vi "FRCts20_WebMethods_Events_Events_GET.vi"(7 "httpRequestID":u32, 11 "view":string) -> ()   [LabVIEW 2014]
doc: "<B>GET</B> on the specified <B>competition</B> resource\n\n<B>Default Return:</B> <B>competition</B> information and list of contained divisions\n\n<B>query =</B> info - Returns only <B>competition</B> information\n stats - Returns statistics for <B>competition</B>\n images - Returns .png and .jpeg images for <B>competition</B>\n videos - Returns .wmv videos for <B>competition</B>\n\nhttp://<server address>:<port>/FRCts/competition/<B>competition</B>"
uses:
  FRCts20_WebMethods.lvlib
  Backend/source/VI Source/FRCts20_Backend_API/FRCts20_Backend_API.lvlib
  <vilib>/wsapi/NI_WebServices.lvlib
  ESP Engine/source/VI Source/FRCts20_EspEngine.lvlib
  Web Method Public Interface/FRCts20_WebMethods_ctl_teamIdentifier.ctl
  Web Method Public Interface/FRCts20_WebMethods_ctl_singleEvent.ctl
  Web Method Public Interface/FRCts20_WebMethods_ctl_events.ctl
  Backend/source/VI Source/FRCts20_Backend_API/FRCts20_Backend_API_Command_Division.ctl
  Backend/source/VI Source/FRCts20_Backend_API/FRCts20_Backend_API_Event.vi
panel:
  in  "events":string
  out "error out":errorcluster
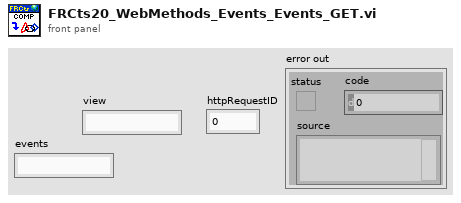
[diagram p1: front panel]
types:
  T1 = typedef "FRCts20_Backend_API.lvlib/FRCts20_Backend_API_Command_Division.ctl" = string
  T2 = typedef "FRCts20_WebMethods.lvlib/FRCts20_WebMethods_ctl_events.ctl" = cluster{"Live Events":cluster{"Team":T3[], "Issue Count":i32, "Location":string, "Start Date ":timestamp}[], "Non Live Events":T4[]}
  T3 = typedef "FRCts20_WebMethods.lvlib/FRCts20_WebMethods_ctl_teamIdentifier.ctl" = cluster{"Team Nickname":string, "Team Number ":u32, "UniqueId":u32}
  T4 = typedef "FRCts20_WebMethods.lvlib/FRCts20_WebMethods_ctl_singleEvent.ctl" = cluster{"Team":T3[], "Issue Count":i32, "Location":string, "Start Date ":timestamp}
  T5 = typedef "FRCts20_WebMethods.lvlib/FRCts20_WebMethods_ctl_returntype.ctl" = string
  T6 = typedef "FRCts20_EspEngine.lvlib/FRCts20_EspEngine_Universe.ctl" = cluster{"TeamsListLength":i16, "Teams":T7[], "LiveEventListLength":i16, "LiveEvents":T12[], "NonLiveEventListLength":i16, "NonLiveEvents":T12[], "OpenIssueCount":i16, "NotFoundStatus":bool}
  T7 = typedef "FRCts20_EspEngine.lvlib/FRCts20_EspEngine_Team.ctl" = cluster{"Team":T8, "RequestListLength":i16, "Requests":T10[]}
  T8 = typedef "FRCts20_WebMethods.lvlib/FRCts20_WebMethods_ctl_singleTeam.ctl" = cluster{"Events":string[], "Robot Name":string, "Kinect":bool, "Vision":bool, "Can":bool, "Tags":string, "Avatar URL":string, "Team":T3, "SWType":T9}
  T9 = typedef "FRCts20_Backend_API.lvlib/FRCts20_Backend_API_SW.ctl" = string
  T10 = typedef "FRCts20_WebMethods.lvlib/FRCts20_WebMethods_ctl_request.ctl" = cluster{"Event":string, "Description":string, "Status":T11, "Open Date":string, "Last Update":string, "Close Date":string, "UniqueId":i32, "Team":cluster{"Team Nickname":string, "Team Number ":i32, "UniqueId":i32}, "Comments":cluster{"Request Number":dbl, "Text":string, "Author":string, "IsSolution":bool, "Team":cluster{"Team Nickname":string, "Team Identifier ":dbl}, "UniqueId":i32}[]}
  T11 = typedef "FRCts20_Backend_API.lvlib/FRCts20_Backend_API_Status.ctl" = enum16{"Open", "In Work", "Closed"}
  T12 = typedef "FRCts20_EspEngine.lvlib/FRCts20_EspEngine_Event.ctl" = cluster{"Single Event":T4, "EventOpenIssueCount":i16, "Requests":cluster{"RequestId":i32, "Request Description":string, "Team Number":i32}[], "ClosedRequests":cluster{"RequestId":i32, "Request Description":string, "Team Number":i32}[], "NotFoundStatus":bool}
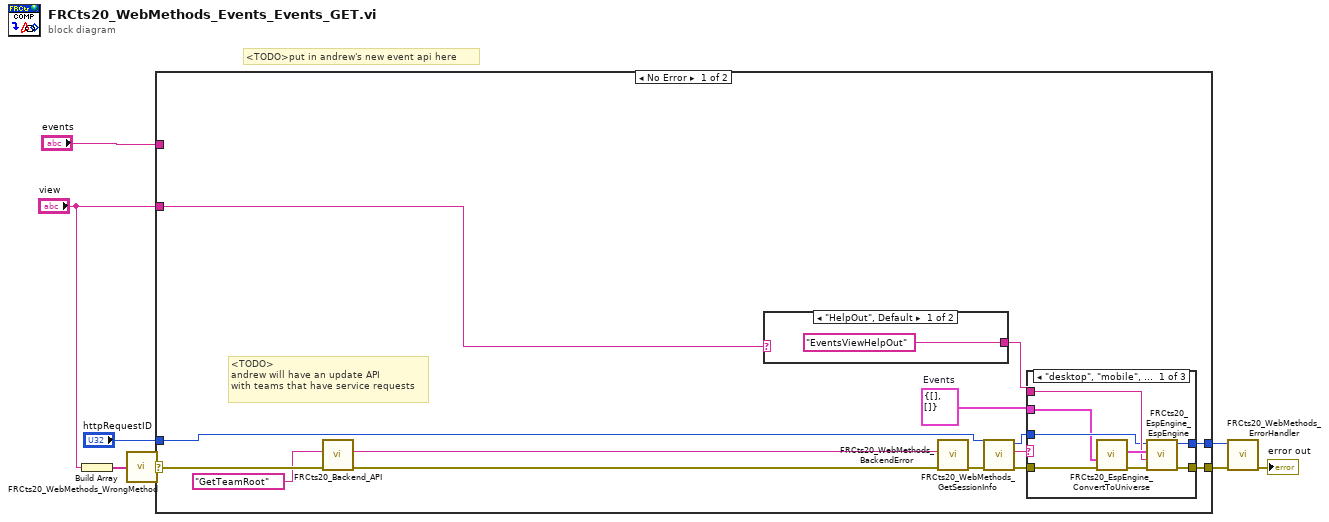
[diagram p0: block diagram]
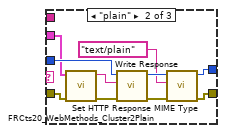
[diagram p2: hidden frame]
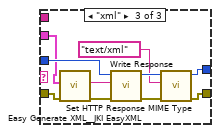
[diagram p3: hidden frame]
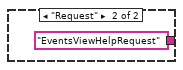
[diagram p4: hidden frame]
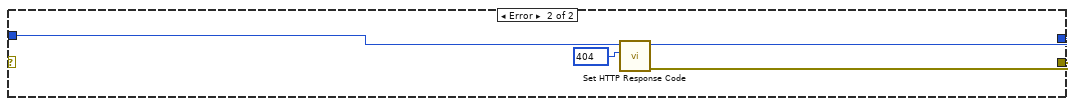
[diagram p5: hidden frame]
diagram:
  # "<TODO>put in andrew's new event api here"
  n1 = Build Array("view") -> (w5:string[])
  n2 = call "FRCts20_WebMethods_WrongMethod.vi"(4:w5) -> (1:w3)  [unwired: 3 in, 1 out]
  n3 = case shown="No Error" w3 {
    selector: w3 -> [w13 _]
    tunnel: "httpRequestID" -> [w19 w56]
    tunnel: [w15 w54] -> w7
    tunnel: [w14 w55] -> w6
    tunnel: "view" -> [w22 _]
    tunnel: "events" -> [_ _]
    frame No Error {
      w10 = T2 {"Live Events"=[], "Non Live Events"=[]}  # Events
      # "<TODO> \nandrew will have an update API\nwith teams that have service requests"
      n4 = call-poly "FRCts20_Backend_API.vi"("error in (no error)"=w13, "Command"=T1 "GetTeamRoot") -> ("error out"=w12:errorcluster, "Status"=w9:string)  [unwired: 7 in, 1 out]
      n5 = case shown="\"HelpOut\", Default" w22 {
        tunnel: ["EventsViewHelpOut" "EventsViewHelpRequest"] -> w18
        frame "HelpOut", Default {
        }
        frame "Request" {
        }
      }
      n6 = call "FRCts20_WebMethods_BackendError.vi"("error in (no error)"=w12, "Status"=w9) -> ("error out"=w17:errorcluster)  [unwired: 8 in, 1 out]
      n7 = call "FRCts20_WebMethods_GetSessionInfo.vi"("error in"=w17, "httpRequestID"=w19) -> ("error out"=w16:errorcluster, "Return Type"=w21:T5, "httpRequestID out"=w20:u32)  [unwired: 7 in]
      n8 = case shown="\"desktop\", \"mobile\", Default" w21 {
        tunnel: w20 -> [w24 w40 w50]
        tunnel: [w25 w37 w44] -> w14
        tunnel: [w26 w36 w45] -> w15
        tunnel: w18 -> [w29 _ _]
        tunnel: w16 -> [w28 w32 w42]
        tunnel: w10 -> [w23 w31 w41]
        frame "desktop", "mobile", Default {
          n9 = call "FRCts20_EspEngine_ConvertToUniverse.vi"("error in (no error)"=w28, "Events"=w23) -> ("error out"=w27:errorcluster, "Universe"=w30:T6)  [unwired: 8 in]
          n10 = call "FRCts20_EspEngine_EspEngine.vi"("error in (no error)"=w27, "Page"=w29, "Cluster"=w30, "httpRequestID"=w24) -> ("error out"=w26:errorcluster, "httpRequestID out"=w25:u32)  [unwired: 6 in]
        }
        frame "plain" {
          n11 = call "FRCts20_WebMethods_Cluster2Plain.vi"("error in (no error)"=w32, "Cluster"=w31) -> ("error out"=w35:errorcluster, "plain text"=w34:string)  [unwired: 8 in]
          n12 = call <vilib>:"Write Response.vi"("error in (no error)"=w35, "response string"=w34, "httpRequestID"=w40) -> ("error out"=w39:errorcluster, "httpRequestID out"=w38:u32)  [unwired: 7 in]
          n13 = call <vilib>:"Set HTTP Response MIME Type.vi"("error in (no error)"=w39, "MIME type (text/html)"="text/plain", "httpRequestID"=w38) -> ("error out"=w36:errorcluster, "httpRequestID out"=w37:u32)  [unwired: 7 in]
        }
        frame "xml" {
          n14 = call <vilib>:"Easy Generate XML__JKI EasyXML.vi"("error in (no error)"=w42, "LabVIEW Data"=w41) -> ("error out"=w49:errorcluster, "XML String"=w48:string)  [unwired: 8 in]
          n15 = call <vilib>:"Write Response.vi"("error in (no error)"=w49, "response string"=w48, "httpRequestID"=w50) -> ("error out"=w46:errorcluster, "httpRequestID out"=w47:u32)  [unwired: 7 in]
          n16 = call <vilib>:"Set HTTP Response MIME Type.vi"("error in (no error)"=w46, "MIME type (text/html)"="text/xml", "httpRequestID"=w47) -> ("error out"=w45:errorcluster, "httpRequestID out"=w44:u32)  [unwired: 7 in]
        }
      }
    }
    frame Error {
      w53 = 404 items=["100"=100, "101"=101, "200"=200, "201"=201, "202"=202, "203"=203, "204"=204, "205"=205, "206"=206, "300"=300, "301"=301, "302"=302, "303"=303, "304"=304, "305"=305, "306"=306, "307"=307, "400"=400, "401"=401, "402"=402, "403"=403, "404"=404, "405"=405, "406"=406, "407"=407, "408"=408, "409"=409, "410"=410, "411"=411, "412"=412, "413"=413, "414"=414, "415"=415, "416"=416, "417"=417, "500"=500, "501"=501, "502"=502, "503"=503, "504"=504, "505"=505] ("response code (200)")
      n17 = call <vilib>:"Set HTTP Response Code.vi"("response code (200)"=w53, "httpRequestID"=w56) -> ("error out"=w54:errorcluster, "httpRequestID out"=w55:u32)  [unwired: 8 in]
    }
  }
  n18 = call "FRCts20_WebMethods_ErrorHandler.vi"("error in"=w7, "httpRequestID"=w6) -> ("error out"=→"error out":errorcluster)  [unwired: 9 in]
